vi "Serialize - JSON.vi"(8 "error in":errorcluster, 11 "PAS Cell Data in":refnum<class "PAS Cell Data.lvclass">) -> (0 "error out":errorcluster, 2 "Serialized JSON":string, 3 "PAS Cell Data out":refnum<class "PAS Cell Data.lvclass">)   [LabVIEW 2016, in "PAS Library.lvlib" / "PAS Cell Data.lvclass"]
uses:
  PAS Cell Data.lvclass
  <vilib>/Analysis/Matrix/Datatypes/RealMatrix.ctl
  PAS Cell Data.lvclass/PAS Cell Data.ctl
  <vilib>/Analysis/Matrix/NI_Matrix.lvlib
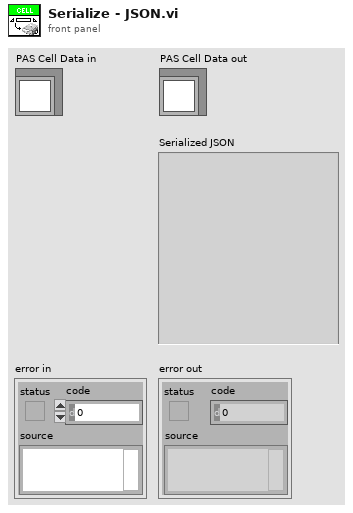
[diagram p1: front panel]
types:
  T1 = typedef "NI_Matrix.lvlib/RealMatrix.ctl" = dbl[][]
  T2 = cluster{"derived":cluster{"f0":sgl, "IA":sgl, "Q":sgl, "max":dbl[], "noiseLim":dbl, "ext":dbl}, "fitData":cluster{"parameters":dbl[], "covariance":T1}, "IABack":dbl, "FittedData":cluster{"Y":sgl[], "dt":dbl}, "MicFreq":cluster{"Y":sgl[], "dt":dbl}, "MicTime":cluster{"Y":i16[], "dt":dbl}, "PhotoDiode":cluster{"Y":i16[], "dt":dbl}, "lRMS":dbl, "phase":cluster{"mic":dbl, "pd":dbl}}
  T3 = cluster{"f0":sgl, "IA":sgl, "Q":sgl, "max":dbl[], "noiseLim":dbl, "abs":dbl}
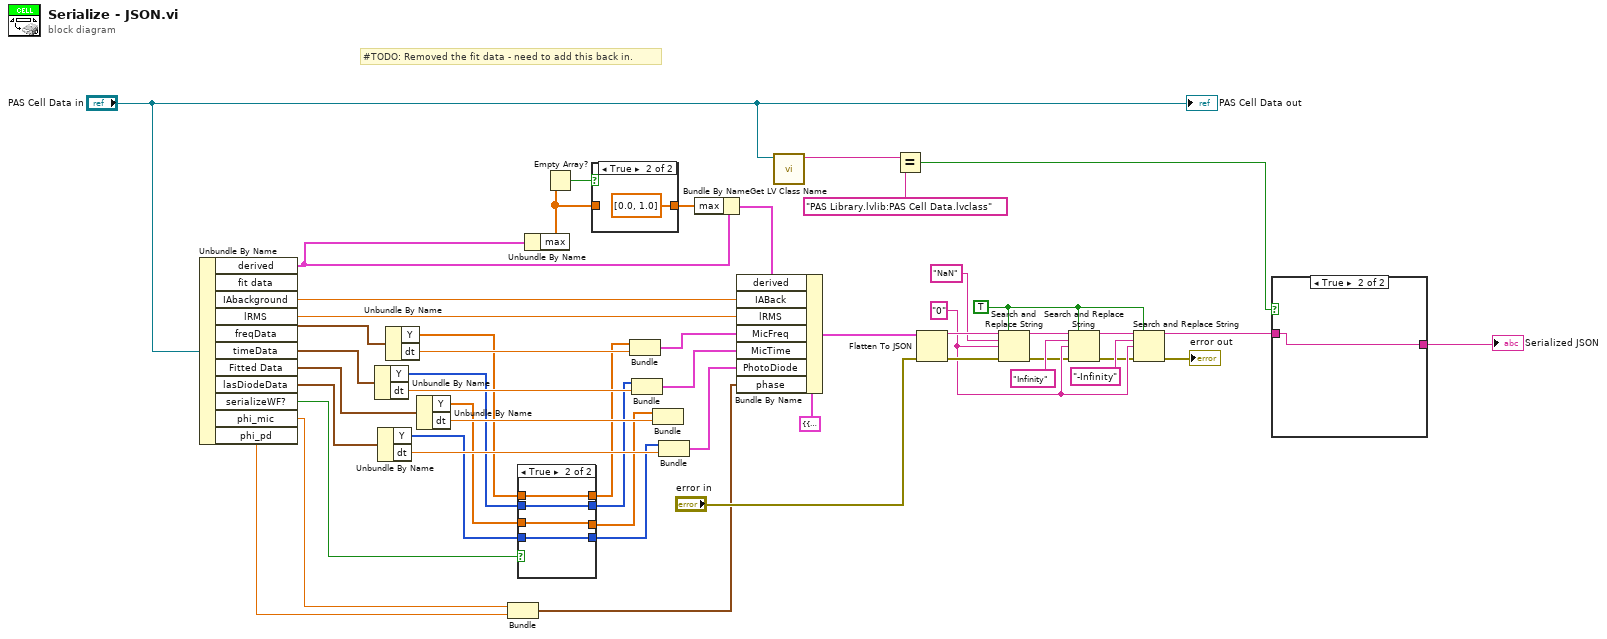
[diagram p0: block diagram]
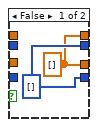
[diagram p2: hidden frame]
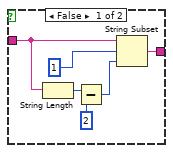
[diagram p4: hidden frame]
diagram:
  w8 = "0" ("replace string (\"\")")
  w6 = TRUE ("replace all? (F)")
  # "#TODO: Removed the fit data - need to add this back in."
  n1 = Unbundle By Name("PAS Cell Data in") -> ("derived"=w28:T3, "IAbackground"=w51:dbl, "lRMS"=w50:dbl, "freqData"=w49:waveform(sgl), "timeData"=w45:waveform(i16), "Fitted Data"=w42:waveform(sgl), "lasDiodeData"=w40:waveform(i16), "serializeWF?"=w24:bool, "phi_mic"=w14:dbl, "phi_pd"=w13:dbl)  [unwired: 1 out]
  n2 = Unbundle By Name(w45) -> ("Y"=w18:i16[], "dt"=w46:dbl)
  n3 = Unbundle By Name(w40) -> ("Y"=w16:i16[], "dt"=w41:dbl)
  n4 = Unbundle By Name(w49) -> ("Y"=w19:sgl[], "dt"=w48:dbl)
  n5 = Unbundle By Name(w42) -> ("Y"=w17:sgl[], "dt"=w43:dbl)
  n6 = Bundle("phi_mic"=w14, "phi_pd"=w13) -> (w12:cluster{"phi_mic":dbl, "phi_pd":dbl})  [unwired: 1 in]
  n7 = case shown="True" w24 {
    tunnel: [w53 w54] -> w23
    tunnel: [w53 w56] -> w22
    tunnel: [w52 w57] -> w21
    tunnel: [w52 w55] -> w20
    tunnel: w19 -> [_ w57]
    tunnel: w18 -> [_ w56]
    tunnel: w17 -> [_ w55]
    tunnel: w16 -> [_ w54]
    frame False {
      w53 = i16[] [] ("Y")
      w52 = sgl[] [] ("Y")
    }
    frame True {
    }
  }
  n8 = Unbundle By Name(w28) -> ("max"=w29:dbl[])
  n9 = Empty Array?(array=w29) -> (empty?=w30:bool)
  n10 = case shown="True" w30 {
    tunnel: w29 -> [w58 _]
    tunnel: [w58 dbl[] [0.0, 1.0] ("max")] -> w27
    frame False {
    }
    frame True {
    }
  }
  n11 = Bundle("Y"=w21, "dt"=w48) -> (w47:cluster{"Y":sgl[], "dt":dbl})  [unwired: 1 in]
  n12 = Bundle("Y"=w22, "dt"=w46) -> (w44:cluster{"Y":i16[], "dt":dbl})  [unwired: 1 in]
  n13 = Bundle("Y"=w20, "dt"=w43) -> ()  [unwired: 1 in, 1 out]
  n14 = Bundle("Y"=w23, "dt"=w41) -> (w39:cluster{"Y":i16[], "dt":dbl})  [unwired: 1 in]
  n15 = Bundle By Name(cluster=w28, "max"=w27) -> (w26:T3)
  n16 = Bundle By Name(cluster=T2 {"derived"={"f0"=0.0, "IA"=0.0, "Q"=0.0, "max"=[0.0], "noiseLim"=0.0, "ext"=0.0}, "fitData"={"parameters"=[0.0], "covariance"=[[0.0, 0.0], [0.0, 0.0]]}, "IABack"=0.0, "FittedData"={"Y"=[0.0], "dt"=0.0}, "MicFreq"={"Y"=[0.0], "dt"=0.0}, "MicTime"={"Y"=[0], "dt"=0.0}, "PhotoDiode"={"Y"=[0], "dt"=0.0}, "lRMS"=0.0, "phase"={"mic"=0.0, "pd"=0.0}}, "derived"=w26, "IABack"=w51, "lRMS"=w50, "MicFreq"=w47, "MicTime"=w44, "PhotoDiode"=w39, "phase"=w12) -> (w38:T2)
  n17 = call <vilib>:"Get LV Class Name.vi"("object"="PAS Cell Data in") -> ("class name"=w34:string)  [unwired: 9 in, 1 out]
  n18 = Equal?(x=w34, y="PAS Library.lvlib:PAS Cell Data.lvclass") -> (x = y?=w1:bool)
  n19 = Flatten To JSON(anything=w38, error in (no error)="error in") -> (JSON string=w37:string, 11:w25:errorcluster)  [unwired: 1 in]
  n20 = Search and Replace String(replace all?=w6, input string=w37, search string="NaN", replace string=w8, error in=w25) -> (result string=w11:string, error out=w4:errorcluster)  [unwired: 3 in, 2 out]
  n21 = Search and Replace String(replace all?=w6, input string=w11, search string="Infinity", replace string=w8, error in=w4) -> (result string=w10:string, error out=w3:errorcluster)  [unwired: 3 in, 2 out]
  n22 = Search and Replace String(replace all?=w6, input string=w10, search string="-Infinity", replace string=w8, error in=w3) -> (result string=w9:string, error out=→"error out":errorcluster)  [unwired: 3 in, 2 out]
  n23 = case shown="True" w1 {
    tunnel: w9 -> [w64 w66]
    tunnel: [w60 w66] -> w32
    frame False {
      n24 = String Length(string=w64) -> (length=w63:i32)
      n25 = Subtract(x=w63, y=2) -> (x-y=w61:i32)
      n26 = String Subset(string=w64, offset (0)=1, length (rest)=w61) -> (substring=w60:string)
    }
    frame True {
    }
  }
  "Serialized JSON" <- w32
  "PAS Cell Data out" <- "PAS Cell Data in"
